vi "FPGA.vi"() -> ()   [LabVIEW 2013]
doc: "This VI implements a 4 channel rising-edge delay generator.\n\nThe time offset of each pulse is configurable. Delay times are specified in FPGA clock ticks.\n\nPulses can be divided, e.g. if the pulse division parameterchannel A has pulse division set to 1, and channel B is set to 2, channel B will fire with every other pulse of channel A."
uses:
  <vilib>/rvi/Emulation/niFpgaSctlEmulationGetInTimedLoop.vi
  <vilib>/rvi/eio/common/nirviEmuTemplateMethod_errors.vi
  <vilib>/rvi/Emulation/niFpgaProcessEmulError.vi
  <vilib>/rvi/Emulation/niFpgaEmulationReportErrorSimple.vi
  <vilib>/rvi/Emulation/niFpgaGetClockAttributes.vi
  <vilib>/rvi/Emulation/niFpgaCriticalErrorInLSC.vi
  <vilib>/eio/EIONode/EIONode.xnode
panel:
  out "Pulse train too long":bool
  in  "Channel A delay":u32
  in  "Channel B delay":u32=200
  in  "Channel C delay":u32=100
  in  "Channel D delay":u32=300
  in  "Channel C pulse divide":u32=1 min=1
  in  "Channel D pulse divide":u32=1 min=1
  in  "Channel B pulse divide":u32=1 min=1
  in  "Channel A pulse divide":u32=1 min=1
  in  "Pulse width (ticks)":u32=800
  in  "Stop":bool
  in  "Channel D on/off":bool=TRUE
  in  "Channel C on/off":bool=TRUE
  in  "Channel B on/off":bool=TRUE
  in  "Channel A on/off":bool=TRUE
  in  "Pulses on/off":bool
  in  "Ticks per cycle":u32=80000
  # "CompactRIO Pulse Generator\n\nDr. Chris Empson\nSchool of Chemistry\nUniversity of Leeds\nUK\n\nc.j.empson@leeds.ac.uk\nTwitter: @monty_mcmont\nDownloaded from https://github.com/mcmont/LabVIEW_examples"
  # "Pulse train settings"
  # "Cycle settings"
  # "WARNING: Setting the correct number of ticks per cycle may be critical to the proper functioning of the connected equipment."
  # "The CompactRIO clock runs at 40MHz, 40 million ticks per second.\n\nTo achieve a cycle time of 500Hz, 'ticks per cycle' should be set \nto 80,000. This is the default value.\n\n1Hz = 40,000,000 ticks per cycle\n10Hz = 4,000,000 ticks per cycle\n250Hz =  160,000 ticks per cycle\n500Hz =    80,000 ticks per cycle\n\nN.B. The number of ticks, rather than the more user-friendly cycle rate in Hz is used in this implementation to save space on the FPGA. If we specified the cycle rate we'd need to divide the number of cycles per second by the cycle rate; division is a very expensive operation on an FPGA!"
  # "Check your equipment's documentation to determine the required pulse width. At 40MHz a pulse width of 20us equates to 800 ticks."
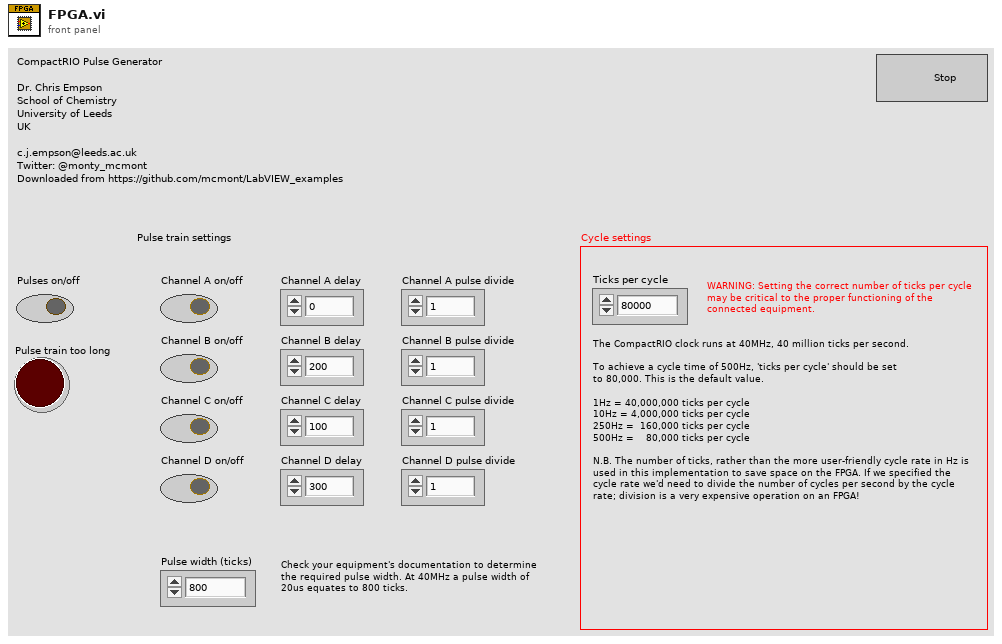
[diagram p1: front panel]
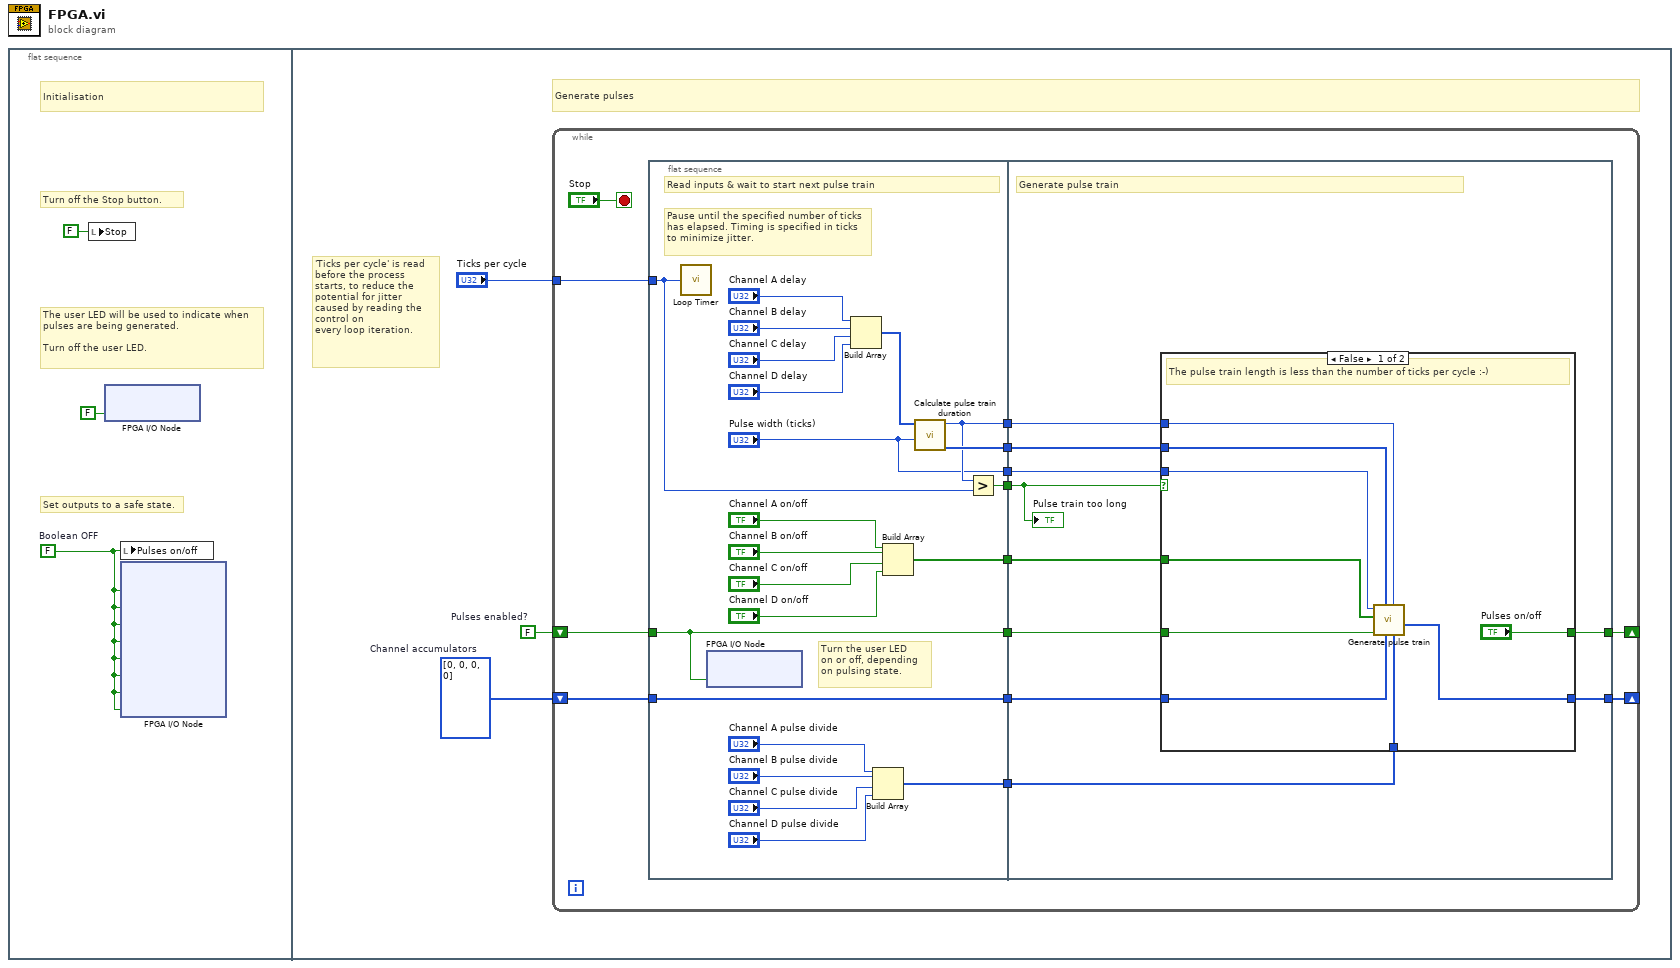
[diagram p0: block diagram]
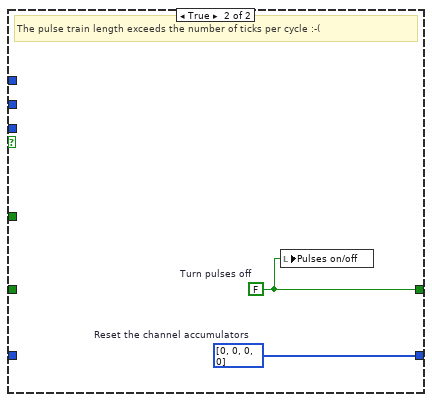
[diagram p2: hidden frame]
diagram:
  n1 = flat-sequence {
    frame #0 {
      w1 = FALSE  # Boolean OFF
      # "Turn off the Stop button."
      # "Initialisation"
      # "The user LED will be used to indicate when pulses are being generated.\n\nTurn off the user LED."
      # "Set outputs to a safe state."
      n2 = local write "Stop"(FALSE ("A")) -> ()
      n3 = xnode "FPGA I/O Node"("FPGA LED"=FALSE) -> ()  [unwired: 1 in, 1 out]
      n4 = local write "Pulses on/off"(w1) -> ()
      n5 = xnode "FPGA I/O Node"("Mod1/DIO0"=w1, "Mod1/DIO1"=w1, "Mod1/DIO2"=w1, "Mod1/DIO3"=w1, "Mod1/DIO4"=w1, "Mod1/DIO5"=w1, "Mod1/DIO6"=w1, "Mod1/DIO7"=w1) -> ()  [unwired: 8 in, 8 out]
    }
    frame #1 {
      w4 = u32[] [0, 0, 0, 0]  # Channel accumulators
      w5 = FALSE  # Pulses enabled?
      # "Generate pulses"
      # "'Ticks per cycle' is read before the process starts, to reduce the potential for jitter caused by reading the control on \nevery loop iteration."
      n6 = while {
        shift-right: [w20] -> _
        shift-left: w5 -> [w14]
        tunnel: "Ticks per cycle" -> [w15]
        shift-right: [w11] -> _
        shift-left: w4 -> [w9]
        stop <- "Stop" stop-if-true
        n7 = flat-sequence {
          tunnel: [w24] -> w19
          tunnel: ["Pulse width (ticks)"] -> w18
          tunnel: [w30] -> w17
          tunnel: [w38] -> w16
          tunnel: w15 -> [w22]
          tunnel: w14 -> [w37]
          tunnel: [w37] -> w13
          tunnel: [w36] -> w10
          tunnel: w9 -> [w31]
          tunnel: [w31] -> w8
          tunnel: [w21] -> w7
          tunnel: [w52] -> w20
          tunnel: w13 -> [w49]
          tunnel: w16 -> [w50]
          tunnel: w17 -> [w51]
          tunnel: w18 -> [w45]
          tunnel: w19 -> [w44]
          tunnel: [w48] -> w11
          tunnel: w10 -> [w47]
          tunnel: w8 -> [w46]
          tunnel: w7 -> [w43]
          frame #0 {
            # "Read inputs & wait to start next pulse train"
            # "Turn the user LED\non or off, depending\non pulsing state."
            # "Pause until the specified number of ticks has elapsed. Timing is specified in ticks to minimize jitter."
            n8 = call "Loop Timer"("Count(Ticks)"=w22) -> ()  [unwired: 1 out]
            n9 = xnode "FPGA I/O Node"("FPGA LED"=w37) -> ()  [unwired: 1 in, 1 out]
            n10 = Build Array("Channel A delay", "Channel B delay", "Channel C delay", "Channel D delay") -> (w25:u32[])
            n11 = Build Array("Channel A pulse divide", "Channel B pulse divide", "Channel C pulse divide", "Channel D pulse divide") -> (w36:u32[])
            n12 = Build Array("Channel A on/off", "Channel B on/off", "Channel C on/off", "Channel D on/off") -> (w38:bool[])
            n13 = call "Calculate pulse train duration.vi"("Pulse width (ticks)"="Pulse width (ticks)", "Channel timings in (ticks)"=w25) -> ("Channel timings out (ticks)"=w30:u32[], "Pulse train length (ticks) out"=w24:u32)  [unwired: 8 in]
            n14 = Greater?(x=w24, y=w22) -> (0:w21:bool)
          }
          frame #1 {
            # "Generate pulse train"
            n15 = case shown="False" w43 {
              tunnel: ["Pulses on/off" w62] -> w52
              tunnel: w51 -> [w60 _]
              tunnel: w50 -> [w59 _]
              tunnel: w49 -> [w58 _]
              tunnel: [w57 w63] -> w48
              tunnel: w47 -> [w56 _]
              tunnel: w46 -> [w55 _]
              tunnel: w45 -> [w54 _]
              tunnel: w44 -> [w53 _]
              frame False {
                # "The pulse train length is less than the number of ticks per cycle :-)"
                n16 = call "Generate pulse train.vi"("Pulse division settings in"=w56, "Pulse train length (ticks) in"=w53, "Channel accumulators in"=w55, "Channel timings (ticks) in"=w60, "Pulses enabled?"=w58, "Channels on/off"=w59, "Pulse width (ticks)"=w54) -> ("Channel accumulators out"=w57:u32[])  [unwired: 4 in]
              }
              frame True {
                w63 = u32[] [0, 0, 0, 0]  # Reset the channel accumulators
                w62 = FALSE  # Turn pulses off
                # "The pulse train length exceeds the number of ticks per cycle :-("
                n17 = local write "Pulses on/off"(w62) -> ()
              }
            }
            "Pulse train too long" <- w43
          }
        }
      }
    }
  }
